vi "UHR-Fleezers Control (host) - 12.1_Jonathan.vi"() -> ()   [LabVIEW 2012] (continued)
      tunnel: w1563 -> [w3002]
      tunnel: w1512 -> [w3001]
      tunnel: w1511 -> [w3000]
      tunnel: w1510 -> [w2999]
      tunnel: w1433 -> [w2998]
      frame #0 {
        n1592 = Or(x="Save N Sets", y="Start Saving") -> (x .or. y?=w2749:bool)
        n1593 = To Double Precision Float(number=w2765) -> (double precision float=w2759:dbl)
        n1594 = Build Array(w2749, "Save Calibration", w2762, w2754) -> (w2764:bool[])
        n1595 = Compound Arithmetic op=OR("Save Calibration", w2762, w2749, w2754) -> (w2767:bool)
        n1596 = Boolean Array To Number(Boolean array=w2764) -> (number=w2761:u32)
        n1597 = feedback #28(FALSE ("Save APD Data\nwith Trap Data")) -> (w2743:bool)
        n1598 = feedback #29(refnum<k0> refnum) -> (w2770:refnum<file>)
        n1599 = feedback #30(refnum<k0> refnum) -> (w2745:refnum<file>)
        n1600 = feedback #31(FALSE ("Save APD Data\nwith Trap Data")) -> (w2753:bool)
        n1601 = feedback #32(refnum<k0> refnum) -> (w2756:refnum<file>)
        n1602 = feedback #33(0) -> (w2772:i32)
        n1603 = feedback #34() -> (w2760:u32)  [unwired: 1 out]
        n1604 = case shown="True" w2767 {
          tunnel: [w2779 1] -> w2768
          tunnel: w2772 -> [w2781 _]
          tunnel: [w2780 w2812] -> w2769
          tunnel: w2770 -> [w2780 _]
          tunnel: w2766 -> [_ w2830]
          tunnel: w2759 -> [_ w2828]
          tunnel: w2761 -> [_ w2831]
          tunnel: [w2778 w2811] -> w2758
          tunnel: w2760 -> [w2778 _]
          tunnel: [w2777 w2809] -> w2755
          tunnel: w2756 -> [w2777 _]
          tunnel: [w2776 w2808] -> w2752
          tunnel: w2753 -> [w2776 _]
          tunnel: "Start Saving" -> [_ w2806]
          tunnel: w2748 -> [_ w2805]
          tunnel: [w2775 w2797] -> w2741
          tunnel: w2745 -> [w2775 _]
          tunnel: [w2774 w2796] -> w2742
          tunnel: w2743 -> [w2774 _]
          frame False {
            n1605 = Increment(x=w2781) -> (x+1=w2779:i32)
          }
          frame True {
            w2802 = FALSE ("Start Saving")
            w2807 = 9.0  # File Version
            w2814 = FALSE ("prepend array or string size? (T)")
            w2813 = T38."big-endian, network order" ("byte order (0:big-endian, network order)")
            n1606 = local read "BD 1 Frequency 1 (MHz)"() -> (w2827:dbl)
            n1607 = local read "BD 2 Frequency 1 (MHz)"() -> (w2826:dbl)
            n1608 = local read "BD 1 Frequency 2 (MHz)"() -> (w2825:dbl)
            n1609 = local read "BD 2 Frequency 2 (MHz)"() -> (w2824:dbl)
            n1610 = local read "BD 1 Frequency 3 (MHz)"() -> (w2823:dbl)
            n1611 = local read "BD 2 Frequency 3 (MHz)"() -> (w2822:dbl)
            n1612 = Array Size(array=w2805) -> (size(s)=w2804:i32)
            n1613 = To Double Precision Float(number=w2804) -> (double precision float=w2803:dbl)
            n1614 = local write "Save Calibration"(w2802) -> ()
            n1615 = local write "Start Saving"(w2802) -> ()
            n1616 = Build Array("Save APD Data\nwith Trap Data", "Save Trap Pos. Data") -> (w2799:bool[])
            n1617 = Boolean Array To Number(Boolean array=w2799) -> (number=w2798:u32)
            n1618 = Build Array(w2827, w2826, w2825, w2824, w2823, w2822) -> (w2821:dbl[])
            n1619 = case shown="1, Default" w2831 {
              tunnel: w2830 -> [w2902 w2922 w2938 w2976]
              tunnel: w2803 -> [w2907 w2929 w2958 w2995]
              tunnel: w2828 -> [w2906 w2928 w2957 w2994]
              tunnel: [w2903 w2924 w2949 w2986] -> w2819
              tunnel: [w2894 "Cal sets to save" w2939 w2977] -> w2811
              tunnel: w2821 -> [w2904 w2925 w2951 w2988]
              tunnel: "Save APD Data\nwith Trap Data" -> [w2901 _ w2935 w2974]
              tunnel: [w2901 w2916 w2935 w2974] -> w2808
              tunnel: w2807 -> [w2897 w2917 w2933 w2972]
              tunnel: w2806 -> [w2896 _ _ _]
              tunnel: [w2887 w2916 w2932 w2962] -> w2796
              tunnel: "Save Trap Pos. Data" -> [w2887 _ w2932 w2962]
              tunnel: w2798 -> [w2886 _ w2931 w2961]
              frame 1, Default {
                # "timeseries"
                n1620 = case shown="True" "Profile" {
                  tunnel: [w2910 w2914] -> w2891
                  tunnel: [w2910 w2913] -> w2890
                  tunnel: [w2910 w2912] -> w2889
                  tunnel: [w2910 w2911] -> w2888
                  frame False {
                    w2910 = 0.0 ("f")
                  }
                  frame True {
                    n1621 = local read "Current Position"() -> (w2915:cluster{dbl, dbl, dbl})
                    n1622 = local read "Y change (mm)"() -> (w2911:dbl)
                    n1623 = Unbundle(w2915) -> (w2914:dbl, w2913:dbl, w2912:dbl)
                  }
                }
                n1624 = local read "Save ave N"() -> (w2909:dbl)
                n1625 = Multiply(x=w2909, y=w2902) -> (x*y=w2908:dbl)
                n1626 = To Double Precision Float(number=w2886) -> (double precision float=w2900:dbl)
                n1627 = Build Array(w2897, w2902, w2908, w2907, w2906, 0.0 ("f")) -> (w2905:dbl[])
                n1628 = Build Array(w2900, w2891, w2890, w2889, w2888) -> (w2898:dbl[])
                n1629 = Select(t=u32 4000000000, s=w2896, f="N sets to save") -> (s? t:f=w2894:u32)
                n1630 = Build Array (concatenate)(w2905, w2904, w2898) -> (w2903:dbl[])
              }
              frame 2 {
                w2919 = 0.0 ("f")
                w2916 = FALSE ("Save APD Data\nwith Trap Data")
                # "calibration"
                n1631 = Boolean To (0,1)(Boolean=w2916) -> (0, 1=w2921:i16)
                n1632 = To Double Precision Float(number=w2921) -> (double precision float=w2920:dbl)
                n1633 = Build Array(w2920, w2919, w2919, w2919, w2919) -> (w2918:dbl[])
                n1634 = Build Array(w2917, w2922, w2922, w2929, w2928, 1.0 ("t")) -> (w2926:dbl[])
                n1635 = Build Array (concatenate)(w2926, w2925, w2918) -> (w2924:dbl[])
                "Calibrating Trap..." <- TRUE ("Calibrating...")
              }
              frame 4 {
                w2936 = 0.0 ("f")
                # "scan dir (x/y = 0/1)"
                # "cycles/step"
                # "n scans (f/b)"
                # "steps"
                # "freq. range"
                # "AOD raster scan"
                n1636 = local read "Number of F/B Scans (AOD)"() -> (w2943:u16)
                n1637 = local read "Cycles/step (AOD)"() -> (w2945:u64)
                n1638 = local read "Scan Range (MHz)"() -> (w2948:dbl)
                n1639 = local read "Scan steps (AOD)"() -> (w2947:u64)
                n1640 = local read "Scan BD"() -> (w2955:bool)
                n1641 = local read "Save ave N"() -> (w2960:dbl)
                n1642 = Boolean To (0,1)(Boolean=w2955) -> (0, 1=w2954:i16)
                n1643 = To Double Precision Float(number=w2943) -> (double precision float=w2942:dbl)
                n1644 = To Double Precision Float(number=w2947) -> (double precision float=w2946:dbl)
                n1645 = To Double Precision Float(number=w2945) -> (double precision float=w2944:dbl)
                n1646 = To Double Precision Float(number=w2954) -> (double precision float=w2953:dbl)
                n1647 = Multiply(x=w2960, y=w2938) -> (x*y=w2959:dbl)
                n1648 = To Double Precision Float(number=w2931) -> (double precision float=w2937:dbl)
                n1649 = Build Array(w2937, w2936, w2936, w2936, w2936) -> (w2934:dbl[])
                n1650 = local read "N sets should be saved"() -> (w2940:dbl)
                n1651 = Build Array(w2953, w2948, w2946, w2944, w2942) -> (w2950:dbl[])
                n1652 = Build Array(w2933, w2938, w2959, w2958, w2957, 2.0 ("t")) -> (w2952:dbl[])
                n1653 = Round Toward +Infinity(x=w2940) -> (ceil(x): smallest int >= x=w2941:dbl)
                n1654 = Build Array (concatenate)(w2952, w2951, w2934, w2950) -> (w2949:dbl[])
                n1655 = To Unsigned Long Integer(number=w2941) -> (unsigned 32bit integer=w2939:u32)
              }
              frame 8 {
                w2969 = 0.0 ("f")
                # "MCL raster scan"
                n1656 = local read "Number of scans (MCL)"() -> (w2964:u64)
                n1657 = local read "Scan lines (y)"() -> (w2963:u64)
                n1658 = local read "2D or 1D Scan"() -> (w2966:bool)
                n1659 = local read "Scan Range (V)\n(of steps)"() -> (w2985:dbl)
                n1660 = local read "Fast Scan Dir"() -> (w2992:bool)
                n1661 = local read "Cycles/step (MCL)"() -> (w2982:u64)
                n1662 = local read "Scan steps (MCL)"() -> (w2984:u64)
                n1663 = Select(t=w2963, s=w2966, f=w2964) -> (s? t:f=w2965:u64)
                n1664 = Boolean To (0,1)(Boolean=w2966) -> (0, 1=w2968:i16)
                n1665 = local read "Save ave N"() -> (w2997:dbl)
                n1666 = local read "Initial X"() -> (w2971:dbl)
                n1667 = local read "Initial Y"() -> (w2970:dbl)
                n1668 = To Double Precision Float(number=w2968) -> (double precision float=w2967:dbl)
                n1669 = Boolean To (0,1)(Boolean=w2992) -> (0, 1=w2991:i16)
                n1670 = To Double Precision Float(number=w2965) -> (double precision float=w2980:dbl)
                n1671 = To Double Precision Float(number=w2984) -> (double precision float=w2983:dbl)
                n1672 = To Double Precision Float(number=w2982) -> (double precision float=w2981:dbl)
                n1673 = To Double Precision Float(number=w2991) -> (double precision float=w2990:dbl)
                n1674 = Multiply(x=w2997, y=w2976) -> (x*y=w2996:dbl)
                n1675 = To Double Precision Float(number=w2961) -> (double precision float=w2975:dbl)
                n1676 = local read "N sets should be saved (MCL)"() -> (w2978:dbl)
                n1677 = Build Array(w2975, w2967, w2969, w2969, w2969) -> (w2973:dbl[])
                n1678 = Build Array(w2990, w2985, w2983, w2981, w2980, w2971, w2970) -> (w2987:dbl[])
                n1679 = Build Array(w2972, w2976, w2996, w2995, w2994, 3.0 ("t")) -> (w2989:dbl[])
                n1680 = Round Toward +Infinity(x=w2978) -> (ceil(x): smallest int >= x=w2979:dbl)
                n1681 = Build Array (concatenate)(w2989, w2988, w2973, w2987) -> (w2986:dbl[])
                n1682 = To Unsigned Long Integer(number=w2979) -> (unsigned 32bit integer=w2977:u32)
              }
            }
            n1683 = local read "Index"() -> (w2836:dbl)
            n1684 = call "Create new save file.vi"("Insert"="", "Ext"=".dat", "Index In"=w2836) -> ("Path Out"=w2794:path, "Index Out"=w2810:dbl)
            n1685 = local write "Save file name"(w2794) -> ()
            n1686 = local write "Index"(w2810) -> ()
            n1687 = local read "connection reference"() -> (w2792:T1)
            n1688 = local write "Save index"(w2810) -> ()
            n1689 = Array Size(array=w2819) -> (size(s)=w2820:i32)
            n1690 = Open/Create/Replace File(file path (use dialog)=w2794, operation (0:open)=T37."create", access (0:read/write)=enum16{"read/write", "read-only", "write-only"}."write-only") -> (refnum out=w2833:refnum<file>)  [unwired: 1 in, 4 out]
            n1691 = local write "Saving..."(TRUE ("Saving...")) -> ()
            n1692 = To Double Precision Float(number=w2820) -> (double precision float=w2818:dbl)
            n1693 = String Length(string="Comment (data description)") -> (length=w2817:i32)
            n1694 = To Double Precision Float(number=w2817) -> (double precision float=w2816:dbl)
            n1695 = Deny Access(7:w2833) -> (3:w2832:refnum<file>)  [unwired: 1 in, 2 out]
            n1696 = Build Array (concatenate)(w2818, w2819, w2816) -> (w2793:dbl[])
            n1697 = case "If fluorescence data to be saved" shown="True" w2808 {
              tunnel: w2794 -> [_ w2885]
              tunnel: [refnum<k0> refnum w2865] -> w2809
              frame False {
              }
              frame True {
                w2864 = 0.0
                n1698 = local read "APD Integration Time (s)"() -> (w2870:dbl)
                n1699 = local read "N APD Samp/step"() -> (w2863:dbl)
                n1700 = Path To String(path=w2885) -> (string=w2884:string)
                n1701 = String Length(string=w2884) -> (length=w2883:i32)
                n1702 = Subtract(x=w2883, y=4) -> (x-y=w2881:i32)
                n1703 = String Subset(string=w2884, length (rest)=w2881) -> (substring=w2880:string)  [unwired: 1 out]
                n1704 = Build Array(w2870, w2863, w2864, w2864, w2864, w2864, w2864, w2864) -> (w2867:dbl[])
                n1705 = Concatenate Strings(w2880, "_fl.dat" ("string")) -> (w2878:string)
                n1706 = Array Size(array=w2867) -> (size(s)=w2869:i32)
                n1707 = String To Path(string=w2878) -> (path=w2874:path)
                n1708 = Open/Create/Replace File(file path (use dialog)=w2874, operation (0:open)=T37."create", access (0:read/write)=enum16{"read/write", "read-only", "write-only"}."write-only") -> (refnum out=w2875:refnum<file>)  [unwired: 1 in, 4 out]
                n1709 = Deny Access(7:w2875) -> (3:w2871:refnum<file>)  [unwired: 1 in, 2 out]
                n1710 = To Double Precision Float(number=w2869) -> (double precision float=w2868:dbl)
                n1711 = Build Array (concatenate)(w2868, w2867) -> (w2866:dbl[])
                n1712 = Write to Binary File(file (use dialog)=w2871, data=w2866, 5:FALSE ("prepend array or string size? (T)"), 9:T38."big-endian, network order" ("byte order (0:big-endian, network order)")) -> (refnum out=w2865:refnum<file>)  [unwired: 1 in, 3 out]
              }
            }
            n1713 = case shown="True" w2796 {
              tunnel: w2794 -> [_ w2847]
              tunnel: [refnum<k0> refnum w2846] -> w2797
              frame False {
              }
              frame True {
                w2842 = 0.0 ("element")
                n1714 = Path To String(path=w2847) -> (string=w2861:string)
                n1715 = Build Array(w2842, w2842, w2842, w2842, w2842, w2842, w2842, w2842) -> (w2843:dbl[])
                n1716 = String Length(string=w2861) -> (length=w2860:i32)
                n1717 = Subtract(x=w2860, y=4) -> (x-y=w2858:i32)
                n1718 = Array Size(array=w2843) -> (size(s)=w2845:i32)
                n1719 = String Subset(string=w2861, length (rest)=w2858) -> (substring=w2857:string)  [unwired: 1 out]
                n1720 = To Double Precision Float(number=w2845) -> (double precision float=w2844:dbl)
                n1721 = Concatenate Strings(w2857, "_pos.dat" ("string")) -> (w2855:string)
                n1722 = Build Array (concatenate)(w2844, w2843) -> (w2841:dbl[])
                n1723 = String To Path(string=w2855) -> (path=w2851:path)
                n1724 = Open/Create/Replace File(file path (use dialog)=w2851, operation (0:open)=T37."create", access (0:read/write)=enum16{"read/write", "read-only", "write-only"}."write-only") -> (refnum out=w2852:refnum<file>)  [unwired: 1 in, 4 out]
                n1725 = Deny Access(7:w2852) -> (3:w2848:refnum<file>)  [unwired: 1 in, 2 out]
                n1726 = Write to Binary File(file (use dialog)=w2848, data=w2841, 5:FALSE ("prepend array or string size? (T)"), 9:T38."big-endian, network order" ("byte order (0:big-endian, network order)")) -> (refnum out=w2846:refnum<file>)  [unwired: 1 in, 3 out]
              }
            }
            n1727 = Write to Binary File(file (use dialog)=w2832, data=w2793, 5:w2814, 9:w2813) -> (refnum out=w2815:refnum<file>)  [unwired: 1 in, 3 out]
            n1728 = Write to Binary File(file (use dialog)=w2815, data="Comment (data description)", 5:w2814, 9:w2813) -> (refnum out=w2812:refnum<file>)  [unwired: 1 in, 3 out]
            n1729 = Bundle("Comment (data description)"="Comment (data description)", "Channel 1 Buffer"="Channel 1 Buffer", "Channel 2 Buffer"="Channel 2 Buffer", "Channel 3 Buffer"="Channel 3 Buffer", "Title"="Title", "DNA Construct"="DNA Construct", "Bead diameter"="Bead diameter", "Name"="Name") -> (w2782:T47)  [unwired: 1 in]
            n1730 = call "MattFileCreator-v9.vi"("Comments"=w2782, "Input Array"=w2793, "File path"=w2794, "table"="labview", "connection reference"=w2792) -> ("connection reference out"=w2791:T1)  [unwired: 5 in, 1 out]
            n1731 = local write "connection reference"(w2791) -> ()
          }
        }
        n1732 = feedback-in #28(w2742) -> ()
        n1733 = feedback-in #29(w2769) -> ()
        n1734 = feedback-in #30(w2741) -> ()
        n1735 = feedback-in #31(w2752) -> ()
        n1736 = feedback-in #32(w2755) -> ()
        n1737 = feedback-in #33(w2768) -> ()
        n1738 = feedback-in #34(w2758) -> ()
      }
      frame #1 {
        n1739 = local read "Saving..."() -> (w3011:bool)
        n1740 = case shown="True" w3011 {
          tunnel: w3015 -> [_ w3026]
          tunnel: w3014 -> [_ w3040]
          tunnel: w3013 -> [_ w3036]
          tunnel: w3012 -> [_ w3035]
          tunnel: w3010 -> [_ w3034]
          tunnel: w3009 -> [_ w3029]
          tunnel: w3008 -> [_ w3028]
          tunnel: w3007 -> [_ w3027]
          tunnel: w3006 -> [_ w3025]
          tunnel: w3005 -> [_ w3023]
          tunnel: w3004 -> [_ w3022]
          tunnel: w3003 -> [_ w3021]
          tunnel: w3002 -> [_ w3020]
          tunnel: w3001 -> [_ w3019]
          tunnel: w3000 -> [_ w3018]
          tunnel: w2999 -> [_ w3017]
          tunnel: w2998 -> [_ w3016]
          frame False {
          }
          frame True {
            n1741 = Multiply(x=w3026, y=w3025) -> (x*y=→"Time (s)":dbl)
            n1742 = Less Or Equal?(x=w3026, y=w3034) -> (x <= y?=w3038:bool)
            n1743 = Or(x="Stop Saving", y="Abort save 2") -> (x .or. y?=w3030:bool)
            n1744 = Not(x=w3030) -> (.not. x?=w3039:bool)
            n1745 = And(x=w3038, y=w3039) -> (x .and. y?=w3037:bool)
            n1746 = case shown="True" w3037 {
              tunnel: w3040 -> [w3047 w3122]
              tunnel: [0.0 w3125] -> w3033
              tunnel: w3026 -> [_ w3123]
              tunnel: w3034 -> [_ w3124]
              tunnel: w3036 -> [_ w3119]
              tunnel: w3035 -> [_ _]
              tunnel: w3029 -> [w3045 w3112]
              tunnel: w3028 -> [w3044 w3113]
              tunnel: w3027 -> [_ w3111]
              tunnel: w3023 -> [_ w3110]
              tunnel: w3022 -> [_ w3054]
              tunnel: w3021 -> [_ w3103]
              tunnel: w3020 -> [_ w3081]
              tunnel: w3019 -> [w3041 w3063]
              tunnel: w3018 -> [w3042 w3062]
              tunnel: w3017 -> [_ w3059]
              tunnel: w3016 -> [_ w3057]
              frame False {
                w3043 = FALSE
                n1747 = Close File(refnum=w3047) -> ()  [unwired: 1 in, 2 out]
                n1748 = case shown="True" w3044 {
                  tunnel: w3045 -> [_ w3049]
                  frame False {
                  }
                  frame True {
                    n1749 = Close File(refnum=w3049) -> ()  [unwired: 1 in, 2 out]
                  }
                }
                n1750 = case shown="True" w3041 {
                  tunnel: w3042 -> [_ w3048]
                  frame False {
                  }
                  frame True {
                    n1751 = Close File(refnum=w3048) -> ()  [unwired: 1 in, 2 out]
                  }
                }
                n1752 = local write "Raster Scanning..."(w3043) -> ()
                n1753 = local write "Calibrating Trap..."(w3043) -> ()
                n1754 = call <vilib>:"Beep.vi"() -> ()  [unwired: 3 in, 9 out]
                n1755 = local write "Stop Saving"(w3043) -> ()
                "Saving..." <- w3043
              }
              frame True {
                n1756 = local read "Calibrating Trap..."() -> (w3114:bool)
                n1757 = case "Write fl. data" shown="True" w3113 {
                  tunnel: w3112 -> [_ w3148]
                  tunnel: w3111 -> [_ w3147]
                  frame False {
                  }
                  frame True {
                    n1758 = Write to Binary File(file (use dialog)=w3148, data=w3147, 5:FALSE ("prepend array or string size? (T)"), 9:T38."big-endian, network order" ("byte order (0:big-endian, network order)")) -> ()  [unwired: 1 in, 4 out]
                  }
                }
                n1759 = Greater?(x="Save ave N", y=1.0) -> (0:w3117:bool)
                n1760 = Not(x=w3114) -> (.not. x?=w3116:bool)
                n1761 = And(x=w3116, y=w3117) -> (x .and. y?=w3060:bool)
                n1762 = case shown="True" w3060 {
                  tunnel: w3059 -> [w3128 w3139]
                  tunnel: [w3128 w3131] -> w3058
                  tunnel: "Save ave N" -> [_ w3132]
                  frame False {
                  }
                  frame True {
                    w3129 = 2 ("dimension size")
                    n1763 = Array Size(array=w3139) -> (size(s)=w3133:i32)
                    n1764 = Divide(x=w3133, y=w3129) -> (x/y=w3137:dbl)
                    n1765 = Reshape Array(w3139, w3137, w3129) -> (w3138:u64[][])
                    n1766 = Transpose 2D Array(2D array=w3138) -> (transposed array=w3136:u64[][])
                    n1767 = for {
                      tunnel: w3136 -> [w3141] mode=indexing
                      tunnel: [w3140] -> w3130 mode=indexing
                      tunnel: w3132 -> [w3142]
                      workers-P: _ -> [_]
                      n1768 = call "downsample 1D array - U64.vi"("Ave N"=w3142, "Array In"=w3141) -> ("Array Out"=w3140:u64[])  [unwired: 1 in]
                    }
                    n1769 = Transpose 2D Array(2D array=w3130) -> (transposed array=w3135:u64[][])
                    n1770 = Divide(x=w3133, y=w3132) -> (x/y=w3134:dbl)
                    n1771 = Reshape Array(w3135, w3134) -> (w3131:u64[])
                  }
                }
                n1772 = case shown="True" w3060 {
                  tunnel: w3119 -> [w3151 w3163]
                  tunnel: [w3151 w3155] -> w3115
                  tunnel: "Save ave N" -> [_ w3156]
                  tunnel: w3110 -> [_ w3154]
                  frame False {
                  }
                  frame True {
                    n1773 = Array Size(array=w3163) -> (size(s)=w3157:i32)
                    n1774 = Array Size(array=w3154) -> (size(s)=w3153:i32)
                    n1775 = Divide(x=w3157, y=w3153) -> (x/y=w3161:dbl)
                    n1776 = Reshape Array(w3163, w3161, w3153) -> (w3162:i16[][])
                    n1777 = Transpose 2D Array(2D array=w3162) -> (transposed array=w3160:i16[][])
                    n1778 = for {
                      tunnel: w3160 -> [w3166] mode=indexing
                      tunnel: [w3165] -> w3152 mode=indexing
                      tunnel: w3156 -> [w3164]
                      workers-P: _ -> [_]
                      n1779 = call "downsample 1D array - I16.vi"("Ave N"=w3164, "Array In"=w3166) -> ("Array Out"=w3165:i16[])  [unwired: 1 out]
                    }
                    n1780 = Transpose 2D Array(2D array=w3152) -> (transposed array=w3159:i16[][])
                    n1781 = Divide(x=w3157, y=w3156) -> (x/y=w3158:dbl)
                    n1782 = Reshape Array(w3159, w3158) -> (w3155:i16[])
                  }
                }
                n1783 = Index Array(array=w3081, index=1) -> (element=w3084:waveform(dbl))
                n1784 = Index Array(array=w3081, index=0) -> (element=w3086:waveform(dbl))
                n1785 = Unbundle By Name(w3084) -> ("Y"=w3088:dbl[])
                n1786 = Unbundle By Name(w3086) -> ("Y"=w3096:dbl[])
                n1787 = case "Write trap pos. data" shown="True" w3063 {
                  tunnel: w3062 -> [_ w3144]
                  tunnel: w3058 -> [_ w3143]
                  frame False {
                  }
                  frame True {
                    n1788 = Write to Binary File(file (use dialog)=w3144, data=w3143, 5:FALSE ("prepend array or string size? (T)"), 9:T38."big-endian, network order" ("byte order (0:big-endian, network order)")) -> ()  [unwired: 1 in, 4 out]
                  }
                }
                n1789 = Write to Binary File(file (use dialog)=w3122, data=w3115, 5:FALSE ("prepend array or string size? (T)"), 9:T38."big-endian, network order" ("byte order (0:big-endian, network order)")) -> ()  [unwired: 1 in, 4 out]
                n1790 = feedback #35(w3088) -> (w3090:dbl[])
                n1791 = Build Array (concatenate)(w3090, w3088) -> (w3089:dbl[])
                n1792 = Select(t=w3088, s=w3054, f=w3089) -> (s? t:f=w3074:dbl[])
                n1793 = feedback-in #35(w3074) -> ()
                n1794 = feedback #36(w3096) -> (w3109:dbl[])
                n1795 = Build Array (concatenate)(w3109, w3096) -> (w3108:dbl[])
                n1796 = Select(t=w3096, s=w3054, f=w3108) -> (s? t:f=w3083:dbl[])
                n1797 = feedback-in #36(w3083) -> ()
                n1798 = Divide(x=w3123, y=w3124) -> (x/y=w3126:dbl)
                n1799 = Multiply(x=w3126, y=100.0) -> (x*y=w3125:dbl)
                n1800 = Build Array(w3083, w3074) -> (→"Saved APD":dbl[][])
                n1801 = Array Size(array=w3083) -> (size(s)=w3101:i32)
                n1802 = Unbundle By Name(w3103) -> ("Y"=w3107:dbl[])
                n1803 = Subtract(x=w3101, y="N pts to average") -> (x-y=w3077:i32)
                n1804 = Multiply(x="N pts to average", y=u16 2) -> (x*y=w3078:u16)
                n1805 = Subtract(x=w3101, y=w3078) -> (x-y=w3076:i32)
                n1806 = feedback #37(w3107) -> (w3106:dbl[])
                n1807 = Build Array (concatenate)(w3106, w3107) -> (w3105:dbl[])
                n1808 = Select(t=w3107, s=w3054, f=w3105) -> (s? t:f=w3104:dbl[])
                "Trap Delta Graph" <- w3104
                n1809 = feedback-in #37(w3104) -> ()
                n1810 = Array Subset(array=w3083, index=w3077, length="N pts to average") -> (w3100:dbl[])
                n1811 = Array Subset(array=w3083, index=w3076, length="N pts to average") -> (w3099:dbl[])
                n1812 = Array Subset(array=w3074, index=w3077, length="N pts to average") -> (w3080:dbl[])
                n1813 = Array Subset(array=w3074, index=w3076, length="N pts to average") -> (w3079:dbl[])
                n1814 = Index Array(array=w3057, index=0) -> (element=w3055:waveform(dbl))
                n1815 = call-poly <vilib>:"Mean.vi"("X"=w3100) -> ("mean"=w3098:dbl)  [unwired: 1 out]
                n1816 = call-poly <vilib>:"Mean.vi"("X"=w3080) -> ("mean"=w3073:dbl)  [unwired: 1 out]
                n1817 = call-poly <vilib>:"Mean.vi"("X"=w3099) -> ("mean"=w3097:dbl)  [unwired: 1 out]
                n1818 = call-poly <vilib>:"Mean.vi"("X"=w3079) -> ("mean"=w3072:dbl)  [unwired: 1 out]
                n1819 = Unbundle By Name(w3055) -> ("Y"=w3052:dbl[])
                n1820 = Subtract(x=w3073, y=w3072) -> (x-y=w3064:dbl)
                "Delta Fl. 2" <- w3064
                n1821 = Subtract(x=w3098, y=w3097) -> (x-y=w3095:dbl)
                "Delta Fl. 1" <- w3095
                n1822 = Initialize Array(w3095, 1 ("dimension size")) -> (w3092:dbl[])
                n1823 = Initialize Array(w3064, 1 ("dimension size")) -> (w3069:dbl[])
                n1824 = feedback #38(w3092) -> (w3093:dbl[])
                n1825 = Build Array (concatenate)(w3093, w3092) -> (w3091:dbl[])
                n1826 = feedback #39(w3069) -> (w3070:dbl[])
                n1827 = Build Array (concatenate)(w3070, w3069) -> (w3068:dbl[])
                n1828 = feedback #40(w3052) -> (w3051:dbl[])
                n1829 = Build Array (concatenate)(w3051, w3052) -> (w3053:dbl[])
                n1830 = Select(t=w3052, s=w3054, f=w3053) -> (s? t:f=w3050:dbl[])
                "Saved trap pos" <- w3050
                n1831 = feedback-in #40(w3050) -> ()
                n1832 = Select(t=w3092, s=w3054, f=w3091) -> (s? t:f=w3067:dbl[])
                n1833 = feedback-in #38(w3067) -> ()
                n1834 = Select(t=w3069, s=w3054, f=w3068) -> (s? t:f=w3066:dbl[])
                n1835 = feedback-in #39(w3066) -> ()
                n1836 = Build Array(w3067, w3066) -> (→"Save APD Deriv":dbl[][])
              }
            }
            "Progress" <- w3033
            "Progress 2" <- w3033
          }
        }
      }
    }
    n1837 = Bundle By Name(cluster=w1683, "Green FB Ch 0"=w1682, "Green FB Ch 1"=w1681) -> (w1661:T46)
    "Green FB Signals (V)" <- w1661
    n1838 = Unbundle By Name(w1661) -> ("Green FB Ch 2"=→"Green FB Plot":dbl)
    n1839 = local read "wait to reset values"() -> (w1752:bool)
    n1840 = Not(x=w1750) -> (.not. x?=w1753:bool)
    n1841 = And(x=w1753, y=w1752) -> (x .and. y?=w1754:bool)
    n1842 = case "Part of MCL raster scanning: returns to initial positions after scan done" shown="True" w1754 {
      tunnel: w1467 -> [w2562 w2569]
      tunnel: [w2562 w2568] -> w1756
      tunnel: w1466 -> [w2561 w2567]
      tunnel: [w2561 w2566] -> w1751
      frame False {
      }
      frame True {
        w2577 = 10.0 ("y")
        w2576 = 32767.0 ("y")
        # "to return scan values\nafter a synchronous \nAOM scan"
        n1843 = local read "AO2"() -> (w2570:dbl)
        n1844 = local read "AO1"() -> (w2571:dbl)
        n1845 = local write "wait to reset values"(FALSE ("wait to reset values")) -> ()
        n1846 = Multiply(x=w2571, y=w2576) -> (x*y=w2573:dbl)
        n1847 = Multiply(x=w2570, y=w2576) -> (x*y=w2575:dbl)
        n1848 = Divide(x=w2573, y=w2577) -> (x/y=w2572:dbl)
        n1849 = Divide(x=w2575, y=w2577) -> (x/y=w2574:dbl)
        n1850 = To Word Integer(number=w2572) -> (16bit integer=w2578:i16)
        n1851 = To Word Integer(number=w2574) -> (16bit integer=w2579:i16)
        n1852 = local read "Total Counts (ticks)"() -> (w2563:u32)
        n1853 = xnode "Read/Write Control"("FPGA VI Reference In"=w2569, "error in"=w2567, "AO1"=w2578, "AO2"=w2579, "MCL count"=w2563) -> ("FPGA VI Reference Out"=w2568:T20, "error out"=w2566:errorcluster)
        n1854 = local read "Scan Range (V)\n(of steps)"() -> (w2564:dbl)
        n1855 = property on="Scan Range (V)\n(of steps)" class="DigNum (strict)"("Val(Sgnl)"=w2564) -> ()  [unwired: 2 in, 2 out]
      }
    }
    n1856 = node-c288() -> ()  [unwired: 2 out]
  }
  n1857 = timed-loop "Control parameters (event loop)" {
    tunnel: w8 -> [w3175]
    shift-right: [w3174] -> _
    shift-left: errorcluster {"status"=FALSE, "code"=0, "source"=""} ("error out") -> [w3173]
    tunnel: [w3172] -> _
    timing: w99 -> [_]
    timing-out: [_] -> w98
    tunnel: w71 -> [w3171]
    tunnel: w12 -> [w3170]
    tunnel: w11 -> [w3169]
    tunnel: w10 -> [w3168]
    tunnel: w9 -> [w3167]
    stop <- w3172 stop-if-true
    n1858 = node-c288() -> ()  [unwired: 2 out]
    n1859 = event shown="[40] \"Index\": Value Change" {
      selector: _ -> [_ _ _ _ _ _ _ _ _ _ _ _ _ _ _ _ _ _ _ _ _ _ _ _ _ _ _ _ _ _ _ _ _ _ _ _ _ _ _ _ _ _ _ _ _ _ _ _ _ _ _ _ _ _ _ _ _ _ _ _ _ _ _ _ _ _ _ _ _ _ _ _ _ _ _ _]
      dyn-events: _ -> [_ _ _ _ _ _ _ _ _ _ _ _ _ _ _ _ _ _ _ _ _ _ _ _ _ _ _ _ _ _ _ _ _ _ _ _ _ _ _ _ _ _ _ _ _ _ _ _ _ _ _ _ _ _ _ _ _ _ _ _ _ _ _ _ _ _ _ _ _ _ _ _ _ _ _ _]
      timeout: _ -> [_ _ _ _ _ _ _ _ _ _ _ _ _ _ _ _ _ _ _ _ _ _ _ _ _ _ _ _ _ _ _ _ _ _ _ _ _ _ _ _ _ _ _ _ _ _ _ _ _ _ _ _ _ _ _ _ _ _ _ _ _ _ _ _ _ _ _ _ _ _ _ _ _ _ _ _]
      tunnel: w3175 -> [w3213 _ _ _ w3251 _ w3273 _ _ _ _ w3339 _ _ w3382 w3388 w3393 w3399 w3435 w3453 w3460 _ w3472 w3476 w3487 w3498 w3509 w3520 w3531 w3542 w3569 w3663 w3670 w3708 _ w3743 w3747 w3758 w3762 w3766 _ w3774 _ _ _ _ _ _ _ _ _ _ _ _ _ _ _ _ _ w4152 _ w4169 _ w4176 w4194 _ w4201 w4209 w4224 w4235 w4241 _ w4250 _ w4269 _]
      tunnel: [w3212 _ _ _ w3241 _ w3272 _ _ w3304 _ w3318 _ _ w3381 w3384 w3390 w3396 w3434 w3451 w3459 _ w3470 _ w3481 w3492 w3503 w3514 w3525 w3536 w3567 w3661 w3668 w3706 _ w3741 w3745 w3748 w3760 w3764 _ w3772 _ _ _ _ _ _ _ _ _ _ _ _ _ _ _ _ _ w4150 _ _ _ _ w4191 _ _ _ _ _ _ _ _ _ _ _] -> w3174
      tunnel: w3173 -> [w3211 _ _ _ w3250 _ w3271 _ _ w3304 _ w3338 _ _ w3380 w3383 w3389 w3395 w3433 w3452 w3458 _ w3471 w3475 w3486 w3497 w3508 w3519 w3530 w3541 w3568 w3662 w3669 w3707 _ w3742 w3746 w3757 w3761 w3765 _ w3773 _ _ _ _ _ _ _ _ _ _ _ _ _ _ _ _ _ w4151 _ w4168 _ w4175 w4193 _ w4200 w4208 w4223 w4234 w4240 _ w4249 _ w4268 _]
      tunnel: [_ _ _ _ _ _ _ _ _ w3303 _ _ _ _ _ _ _ _ _ _ _ _ _ _ _ _ _ _ _ _ _ _ _ _ _ _ _ _ _ _ _ _ _ _ _ _ _ _ _ _ _ _ _ _ _ _ _ _ _ _ _ _ _ _ _ _ _ _ _ _ _ _ _ _ _ _] -> w3172
      tunnel: [_ _ _ _ _ _ _ "Round T1 X" _ _ _ _ _ _ _ _ _ _ _ _ _ _ _ _ _ _ _ _ _ _ _ _ _ _ _ _ _ _ _ _ _ _ _ _ _ _ _ _ _ _ _ _ _ _ _ _ _ _ _ _ _ _ _ _ _ _ _ _ _ _ _ _ _ _ _ _] -> _
      tunnel: [_ _ _ "Adjust Scale\nto Mean" _ _ _ _ _ _ _ _ _ _ _ _ _ _ _ _ _ _ "Test ttrig" _ _ _ _ _ _ _ _ _ _ _ _ _ _ _ _ _ _ _ _ _ _ _ _ _ _ "Flush Sample" "Flush Pump 3" "Flush Pump 1" "Clear Volume" _ _ _ _ _ _ _ _ _ _ _ _ _ _ _ _ _ _ _ _ _ _ _] -> _
      tunnel: [_ _ _ _ _ _ _ _ "Round T2 X" _ "Delayed Interlace Start" _ _ _ _ _ _ _ _ _ _ _ _ _ _ _ _ _ _ _ _ _ _ _ _ _ _ _ _ _ _ _ _ _ _ _ _ _ _ _ _ _ _ _ _ _ _ _ _ _ _ _ _ _ _ _ _ _ _ _ _ _ _ _ _ _] -> _
      tunnel: w3171 -> [_ _ _ _ _ _ _ _ _ _ _ _ _ _ _ _ _ _ _ _ _ _ _ _ _ _ _ _ _ _ _ _ _ _ _ _ _ _ _ _ _ _ _ _ _ w3931 w3938 w3945 w3950 w3959 _ _ w4065 _ _ _ _ _ _ _ _ _ _ _ _ _ _ _ _ _ _ _ _ _ _ _]
      tunnel: w3170 -> [_ _ _ _ _ _ _ _ _ _ _ _ _ _ _ _ _ _ _ _ _ _ _ _ _ _ _ _ _ _ _ _ _ _ _ _ _ _ _ _ _ _ _ w3848 _ _ _ _ _ _ w4003 _ _ w4071 _ w4080 _ w4094 _ _ _ _ _ _ _ _ _ _ _ _ _ _ _ _ _ _]
      tunnel: w3169 -> [_ _ _ _ _ _ _ _ _ _ _ _ _ _ _ _ _ _ _ _ _ _ _ _ _ _ _ _ _ _ _ _ _ _ _ _ _ _ _ _ _ _ _ _ _ _ _ _ _ _ _ _ _ _ _ _ _ _ _ _ _ _ _ _ _ _ _ _ _ _ _ _ _ _ _ _]
      tunnel: w3168 -> [_ _ _ _ _ _ _ _ _ _ _ _ _ _ _ _ _ _ _ _ _ _ _ _ _ _ _ _ _ _ _ _ _ _ _ _ _ _ _ _ _ _ w3785 _ _ _ _ _ _ _ _ w4033 _ _ w4076 _ w4087 _ w4119 _ _ _ _ _ _ _ _ _ _ _ _ _ _ _ _ _]
      tunnel: w3167 -> [_ _ _ _ _ _ _ _ _ _ _ _ _ _ _ _ _ _ _ _ _ _ _ _ _ _ _ _ _ _ _ _ _ _ _ _ _ _ _ _ _ _ _ _ _ _ _ _ _ _ _ _ _ _ _ _ _ _ _ _ _ _ _ _ _ _ _ _ _ _ _ _ _ _ _ _]
      event "AI Count (ticks)", "Sets to FIFO (Traps)", "Save ave N", "FPGA Ave.", "# Samples/channel", "N sets to save": Value Change {
        # "So that if 'Save ave N' is updated, the AOD scanning code updates too."
        n1860 = event-data() -> ()  [unwired: 6 out]
        n1861 = local read "AI Count (ticks)"() -> (w3193:u32)
        n1862 = Boolean To (0,1)(Boolean="Sets to FIFO (Traps)") -> (0, 1=w3203:cluster{"Set 1":i16, "Set 2":i16, "Set 3":i16})
        n1863 = xnode "Read/Write Control"("FPGA VI Reference In"=w3213, "error in"=w3211, "ai count"=w3193, "AI1 Sets to FIFO"="Sets to FIFO (Traps)", "N of AI1 Int Acq Sets"="N Acq Sets (Traps + Fl.)") -> ("error out"=w3212:errorcluster)  [unwired: 1 out]
        n1864 = Cluster To Array(cluster=w3203) -> (array=w3202:i16[])
        n1865 = To Unsigned Long Integer(number=w3202) -> (unsigned 32bit integer=w3182:u32[])
        n1866 = local read "Scan steps (AOD)"() -> (w3204:u64)
        n1867 = Multiply(x=w3193, y="N Acq Sets (Traps + Fl.)") -> (x*y=w3191:u32)
        n1868 = Divide(x=40000000.0, y=w3193) -> (x/y=w3185:dbl)
        "AI rate (Hz)" <- w3185
        "Ave. Rate (Hz)" <- w3185
        n1869 = Add Array Elements(numeric array=w3182) -> (sum=w3194:u32)
        "Trap Sets" <- w3194
        n1870 = Reciprocal(x=w3185) -> (1/x=→"Ave. Period (s)":dbl)
        n1871 = property on="Scan steps (AOD)" class="DigNum (strict)"("Val(Sgnl)"=w3204) -> ()  [unwired: 2 in, 2 out]
        n1872 = Divide(x=w3185, y="N Acq Sets (Traps + Fl.)") -> (x/y=w3208:dbl)
        "Data Rate (Hz)" <- w3208
        n1873 = Reciprocal(x=w3208) -> (1/x=→"Data Period (s)":dbl)
        n1874 = local read "Save ave N"() -> (w3207:dbl)
        n1875 = Divide(x=w3208, y=w3207) -> (x/y=w3206:dbl)
        "Save Data Rate (Hz)" <- w3206
        n1876 = Reciprocal(x=w3206) -> (1/x=→"Save Data Period (s)":dbl)
        n1877 = Multiply(x=w3191, y="# Samples/trap") -> (x*y=w3189:u32)
        "Counts/DMA" <- w3189
        n1878 = property on="Trap Disp. Downsample" class="DigNum (strict)"("Maximum"="# Samples/trap") -> ()  [unwired: 2 in, 2 out]
        n1879 = Multiply(x=w3194, y="# Samples/trap") -> (x*y=w3183:u32)
        "# Samples/channel" <- w3183
        n1880 = Multiply(x=w3183, y=u32 8) -> (x*y=→"Trap AI Elements/DMA read":u32)
        n1881 = local read "APD Int. Count"() -> (w3190:u32)
        n1882 = Multiply(x=w3183, y=u32 3) -> (x*y=→"Trap Pos Elements/DMA read":u32)
        n1883 = Divide(x=w3189, y=w3190) -> (x/y=w3180:dbl)
        "APD Samples/FIFO Acq." <- w3180
        n1884 = Divide(x=w3189, y=40000000.0) -> (x/y=w3187:dbl)
        "DMA Update Period (s)" <- w3187
        n1885 = Multiply(x=2.0, y=w3180) -> (x*y=→"APD Elements/DMA read":dbl)
        n1886 = property on="APD Disp. Downsample" class="DigNum (strict)"("Maximum"=w3180) -> ()  [unwired: 2 in, 2 out]
        n1887 = local read "N sets to save"() -> (w3200:u32)
        n1888 = Multiply(x=w3187, y=w3200) -> (x*y=→"Total Time (s) 2":dbl)
        "FPGA Averaging" <- FALSE ("FPGA Averaging")
      }
      event "Remove Offset": Value Change {
        n1889 = event-data() -> ()  [unwired: 7 out]
        n1890 = local write "Remove Offset"(FALSE ("Remove Offset")) -> ()
        n1891 = local read "Bead Mean (nm)"() -> (w3215:dbl)
        n1892 = local read "Offset (nm)"() -> (w3216:dbl)
        n1893 = Add(x=w3215, y=w3216) -> (x+y=w3214:dbl)
        n1894 = local write "Offset (nm)"(w3214) -> ()
        n1895 = disable-structure shown="Disabled" {
          frame Disabled {
            n1896 = local read "Bead Mean (nm)"() -> (w3221:dbl)
            n1897 = Add(y=w3221) -> (x=w3220:dbl, x+y=w3219:dbl)
            n1898 = Subtract(x=w3221, y=w3220) -> (x-y=w3218:dbl)
            n1899 = property on="Bead Separation" class="WFChart (strict)"("YScale.Minimum"=w3218) -> ()  [unwired: 2 in, 2 out]
            n1900 = property on="Bead Separation" class="WFChart (strict)"("YScale.Maximum"=w3219) -> ()  [unwired: 2 in, 2 out]
          }
          frame Enabled {
          }
        }
      }
      event "Detector Type": Value Change {
        n1901 = event-data() -> ()  [unwired: 7 out]
        n1902 = local read "AI labels"() -> (w3222:string[])
        n1903 = property on="High Res. Display" class="Ring (strict)"("Strings []"=w3222) -> ()  [unwired: 2 in, 2 out]
        n1904 = Build Array (concatenate)(w3222, "none") -> (w3223:string[])
        n1905 = property on="FFT 1 Choice 1" class="Ring (strict)"("Strings []"=w3223) -> ()  [unwired: 2 in, 2 out]
        n1906 = property on="FFT 1 Choice 2" class="Ring (strict)"("Strings []"=w3223) -> ()  [unwired: 2 in, 2 out]
        n1907 = property on="FFT 2 Choice 1" class="Ring (strict)"("Strings []"=w3223) -> ()  [unwired: 2 in, 2 out]
        n1908 = property on="FFT 2 Choice 2" class="Ring (strict)"("Strings []"=w3223) -> ()  [unwired: 2 in, 2 out]
        n1909 = Bundle("APD 1", "APD 2") -> (w3226:cluster{string, string})  [unwired: 1 out]
        n1910 = Cluster To Array(cluster=w3226) -> (array=w3224:string[])
        n1911 = Build Array (concatenate)(w3224, w3223) -> (w3228:string[])
        n1912 = Array Size(array=w3228) -> (size(s)=w3229:i32)
        n1913 = property on="Signals to Plot" class="LstBox (strict)"("Item Names"=w3228) -> ()  [unwired: 2 in, 2 out]
        n1914 = property on="Signals to Plot" class="LstBox (strict)"("Number of Rows"=w3229) -> ()  [unwired: 2 in, 2 out]
        n1915 = property on="All Signals" class="WFChart (strict)"("LegNumRows"=w3229) -> ()  [unwired: 2 in, 2 out]
      }
      event "Adjust Scale\nto Mean": Value Change {
        n1916 = event-data() -> ()  [unwired: 7 out]
        n1917 = local read "APD 1 Rate (Hz)"() -> (w3238:dbl)
        n1918 = Multiply(x=1000.0, y="Above (kHz)") -> (x*y=w3236:dbl)
        n1919 = Multiply(x=1000.0, y="Below (kHz)") -> (x*y=w3234:dbl)
        n1920 = Add(x=w3236, y=w3238) -> (x+y=w3231:dbl)
        n1921 = Subtract(x=w3238, y=w3234) -> (x-y=w3232:dbl)
        n1922 = property on="APD Chart" class="WFChart (strict)"("YScale.Minimum"=w3232) -> ()  [unwired: 2 in, 2 out]
        n1923 = property on="APD Chart" class="WFChart (strict)"("YScale.Maximum"=w3231) -> ()  [unwired: 2 in, 2 out]
      }
      event "Phase adj. (AI1)", "+ phase (AI1)", "- phase (AI1)": Value Change {
        n1924 = event-data() -> ()  [unwired: 7 out]
        n1925 = Negate(x="Phase adj. (AI1)") -> (-x=w3248:i16)
        n1926 = Select(t=w3248, s="- phase (AI1)", f="Phase adj. (AI1)") -> (s? t:f=w3247:i16)
        n1927 = xnode "Read/Write Control"("FPGA VI Reference In"=w3251, "error in"=w3250, "Phase count adjustment"=w3247) -> ("FPGA VI Reference Out"=w3246:T20, "error out"=w3245:errorcluster)
        n1928 = Or(x="- phase (AI1)", y="+ phase (AI1)") -> (x .or. y?=w3242:bool)
        n1929 = xnode "Read/Write Control"("FPGA VI Reference In"=w3246, "error in"=w3245, "+ phase"=w3242) -> ("error out"=w3241:errorcluster)  [unwired: 1 out]
      }
      event "Signals to Plot": Double Click {
        w3254 = u32 9868950 ("Color Box")
        n1930 = event-data() -> ("Row"=w3256:i32)  [unwired: 9 out]
        n1931 = property on="All Signals" class="WFChart (strict)"("Active Plot"=w3256) -> (error out=w3267:errorcluster)  [unwired: 2 in, 1 out]
        n1932 = property on="All Signals" class="WFChart (strict)" props=["Plot", "Visible?", "Plot", "Plot Color"](error in=w3267) -> (error out=w3266:errorcluster, "Plot.Visible?"=w3265:bool)  [unwired: 1 in, 2 out]
        n1933 = Select(t=FALSE ("Plot.Visible"), s=w3265, f=TRUE ("Plot.Visible")) -> (s? t:f=w3260:bool)
        n1934 = property on="All Signals" class="WFChart (strict)"(error in=w3266, "Plot.Visible?"=w3260) -> (error out=w3262:errorcluster)  [unwired: 1 in, 1 out]
        n1935 = property on="All Signals" class="WFChart (strict)"(error in=w3262) -> (error out=w3257:errorcluster, "Plot.Plot Color"=w3261:u32)  [unwired: 1 in, 1 out]
        n1936 = property on="Signals to Plot" class="LstBox (strict)"(error in=w3257, "Active Row"=w3256) -> (error out=w3255:errorcluster)  [unwired: 1 in, 1 out]
        n1937 = Select(t=w3261, s=w3260, f=u32 0) -> (s? t:f=w3258:u32)
        n1938 = property on="Signals to Plot" class="LstBox (strict)"(error in=w3255, "CellFontColor"=w3258, "SelColor"=w3254, "CellBG"=w3254, "CellFontSize"=u32 20 ("Active Row:Cell Font:Size"), "CellFontBold"=TRUE ("Active Row:Cell Font:Bold")) -> ()  [unwired: 1 in, 2 out]
      }
      event "BD 1 Frequency 1 (MHz)", "BD 1 Frequency 2 (MHz)", "BD 1 Frequency 3 (MHz)", "BD 2 Frequency 1 (MHz)", "BD 2 Frequency 2 (MHz)", "BD 2 Frequency 3 (MHz)", "Trap Delta (MHz)": Value Change {
        n1939 = event-data() -> ("CtlRef"=w3270:refnum<vi>)  [unwired: 6 out]
        n1940 = control-ref of="Trap Delta (MHz)"() -> (w3269:refnum<vi>)
        n1941 = Equal?(x=w3269, y=w3270) -> (x = y?=w3268:bool)
        n1942 = case shown="False" "Oscillate Set 1" {
          tunnel: w3273 -> [w3293 _]
          tunnel: [w3292 w3296] -> w3272
          tunnel: w3271 -> [w3291 w3296]
          tunnel: w3268 -> [w3276 _]
          frame False {
            n1943 = local read "BD 1 Frequency 2 (MHz)"() -> (w3280:dbl)
            n1944 = local read "BD 1 Frequency 1 (MHz)"() -> (w3278:dbl)
            n1945 = Subtract(x=w3280, y="Trap Delta (MHz)") -> (x-y=w3277:dbl)
            n1946 = Select(t=w3277, s=w3276, f=w3278) -> (s? t:f=w3275:dbl)
            n1947 = local read "Y RF Frequency Limits (MHz)"() -> (w3281:T17)
            n1948 = local read "X RF Frequency Limits (MHz)"() -> (w3282:T17)
            n1949 = local read "BD 1 Frequency 3 (MHz)"() -> (w3294:dbl)
            n1950 = local write "BD 1 Frequency 1 (MHz)"(w3275) -> ()
            n1951 = local read "BD 2 Frequency 1 (MHz)"() -> (w3285:dbl)
            n1952 = local read "BD 2 Frequency 2 (MHz)"() -> (w3284:dbl)
            n1953 = local read "BD 2 Frequency 3 (MHz)"() -> (w3295:dbl)
            n1954 = call "set RF board frequency - interlace.vi"("Board 2 Frequency Limits"=w3281, "Board 1 Frequency Limits"=w3282, "error in"=w3291, "FPGA VI Reference In"=w3293, "Board 2 Frequency 3 (MHz)"=w3295, "Board 1 Frequency 3 (MHz)"=w3294, "Board 2 Frequency 2 (MHz)"=w3284, "Board 2 Frequency 1 (MHz)"=w3285, "Board 1 Frequency 2 (MHz)"=w3280, "Board 1 Frequency 1  (MHz)"=w3275) -> ("error out"=w3292:errorcluster)  [unwired: 1 out]
            n1955 = Subtract(x=w3285, y=w3284) -> (x-y=w3289:dbl)
            n1956 = Subtract(x=w3275, y=w3280) -> (x-y=w3290:dbl)
            n1957 = Square(x=w3289) -> (x^2=w3287:dbl)
            n1958 = Square(x=w3290) -> (x^2=w3288:dbl)
            n1959 = Add(x=w3288, y=w3287) -> (x+y=w3286:dbl)
            n1960 = Square Root(x=w3286) -> (sqrt(x)=w3283:dbl)
            n1961 = local write "Trap Delta (MHz)"(w3283) -> ()
            n1962 = property on="Initial delta (MHz)" class="DigNum (strict)"("Val(Sgnl)"=w3283) -> ()  [unwired: 2 in, 2 out]
          }
          frame True {
          }
        }
      }
      event "Round T1 X": Value Change {
        n1963 = event-data() -> ()  [unwired: 7 out]
        n1964 = local read "BD 1 Frequency 1 (MHz)"() -> (w3299:dbl)
        n1965 = Round To Nearest(number=w3299) -> (nearest integer value=w3298:dbl)
        n1966 = property on="BD 1 Frequency 1 (MHz)" class="DigNum (strict)"("Val(Sgnl)"=w3298) -> ()  [unwired: 2 in, 2 out]
      }
      event "Round T2 X": Value Change {
        n1967 = event-data() -> ()  [unwired: 7 out]
        n1968 = local read "BD 1 Frequency 2 (MHz)"() -> (w3301:dbl)
        n1969 = Round To Nearest(number=w3301) -> (nearest integer value=w3300:dbl)
        n1970 = property on="BD 1 Frequency 2 (MHz)" class="DigNum (strict)"("Val(Sgnl)"=w3300) -> ()  [unwired: 2 in, 2 out]
      }
      event "Stop All": Value Change {
        n1971 = event-data() -> ()  [unwired: 7 out]
        n1972 = local read "Stop All"() -> (w3303:bool)
      }
      event "Delayed Interlace Start": Value Change {
        n1973 = event-data() -> ()  [unwired: 7 out]
        n1974 = flat-sequence {
          frame #0 {
            n1975 = Multiply(x="Delay to Interlace (s)", y=1000.0) -> (x*y=w3306:dbl)
            n1976 = Wait (ms)(milliseconds to wait=w3306) -> ()  [unwired: 1 out]
          }
          frame #1 {
            n1977 = property on="Green laser mode" class="RadioBtnsControl (strict)"("Val(Sgnl)"=enum32{"Laser ON", "Laser OFF", "Interlace"}."Interlace" ("Value (Signaling)")) -> ()  [unwired: 2 in, 2 out]
          }
        }
      }
      event "BD 1 Amplitude 1 (%)", "BD 1 Amplitude 2 (%)", "BD 1 Amplitude 3 (%)", "BD 2 Amplitude 1 (%)", "BD 2 Amplitude 2 (%)", "BD 2 Amplitude 3 (%)", "Trap 1 ON", "Trap 2 ON", "Trap 3 ON", "Feedback On/Off", "All FB On/Off": Value Change {
        w3330 = i16 1 ("f")
        n1978 = event-data() -> ()  [unwired: 7 out]
        n1979 = local write "Trap 1 (ON/OFF)"("Trap 1 ON") -> ()
        n1980 = local write "Trap 2 (ON/OFF)"("Trap 2 ON") -> ()
        n1981 = Boolean To (0,1)(Boolean="Trap 3 ON") -> (0, 1=w3331:i16)
        n1982 = Boolean To (0,1)(Boolean="Trap 1 ON") -> (0, 1=w3332:i16)
        n1983 = Boolean To (0,1)(Boolean="Trap 2 ON") -> (0, 1=w3333:i16)
        n1984 = Select(t=w3333, s="Trap ON/OFF X or Y Amp?", f=w3330) -> (s? t:f=w3328:i16)
        n1985 = Select(t=w3332, s="Trap ON/OFF X or Y Amp?", f=w3330) -> (s? t:f=w3329:i16)
        n1986 = Select(t=w3331, s="Trap ON/OFF X or Y Amp?", f=w3330) -> (s? t:f=w3327:i16)
        n1987 = Select(t=w3330, s="Trap ON/OFF X or Y Amp?", f=w3333) -> (s? t:f=w3325:i16)
        n1988 = Select(t=w3330, s="Trap ON/OFF X or Y Amp?", f=w3332) -> (s? t:f=w3326:i16)
        n1989 = Select(t=w3330, s="Trap ON/OFF X or Y Amp?", f=w3331) -> (s? t:f=w3324:i16)
        n1990 = And(x="All FB On/Off", y="Feedback On/Off") -> (x .and. y?=w3322:cluster{"Set 1":bool, "Set 2":bool})
        n1991 = local read "BD 1 Amplitude 1 (%)"() -> (w3342:dbl)
        n1992 = local read "BD 1 Amplitude 2 (%)"() -> (w3341:dbl)
        n1993 = local read "BD 1 Amplitude 3 (%)"() -> (w3340:dbl)
        n1994 = Unbundle By Name(w3322) -> ("Set 1"=w3317:bool, "Set 2"=w3314:bool)
        n1995 = local read "Y RF Amplitude Limits (%)"() -> (w3310:T17)
        n1996 = local read "X RF Amplitude Limits (%)"() -> (w3311:T17)
        n1997 = local read "BD 2 Amplitude 1 (%)"() -> (w3343:dbl)
        n1998 = local read "BD 2 Amplitude 2 (%)"() -> (w3344:dbl)
        n1999 = local read "BD 2 Amplitude 3 (%)"() -> (w3345:dbl)
        n2000 = And(x="Trap 2 ON", y=w3314) -> (x .and. y?=w3312:bool)
        n2001 = And(x="Trap 1 ON", y=w3317) -> (x .and. y?=w3315:bool)
        n2002 = Multiply(x=w3329, y=w3342) -> (x*y=w3337:dbl)
        n2003 = Multiply(x=w3341, y=w3328) -> (x*y=w3335:dbl)
        n2004 = Multiply(x=w3340, y=w3327) -> (x*y=w3336:dbl)
        n2005 = Multiply(x=w3343, y=w3326) -> (x*y=w3346:dbl)
        n2006 = Multiply(x=w3344, y=w3325) -> (x*y=w3347:dbl)
        n2007 = Multiply(x=w3345, y=w3324) -> (x*y=w3348:dbl)
        n2008 = call "set RF board amplitude - interlace.vi"("Board 2 Amplitude Limits"=w3310, "Board 1 Amplitude Limits"=w3311, "error in"=w3338, "FPGA VI Reference In"=w3339, "Board 2 Amplitude 3 (%)"=w3348, "Board 1 Amplitude 3 (%)"=w3336, "Board 2 Amplitude 2 (%)"=w3347, "Board 2 Amplitude 1 (%)"=w3346, "Board 1 Amplitude 2 (%)"=w3335, "Board 1 Amplitude 1 (%)"=w3337) -> ("error out"=w3319:errorcluster, "FPGA VI Reference Out"=w3320:T20)
        n2009 = xnode "Read/Write Control"("FPGA VI Reference In"=w3320, "error in"=w3319, "FB On/Off Set 1"=w3315, "FB On/Off Set 2"=w3312) -> ("error out"=w3318:errorcluster)  [unwired: 1 out]
      }
      event "Load parameters": Value Change {
        n2010 = event-data() -> ()  [unwired: 7 out]
        n2011 = property on="Saved AOD Raster Scan Parameter Sets" class="Arr (strict)"() -> ("Index Values"=w3359:u32[])  [unwired: 2 in, 2 out]
        n2012 = Index Array(array=w3359, index=0) -> (element=w3356:u32)
        n2013 = local write "Load parameters"(FALSE ("Load parameters")) -> ()
        n2014 = Index Array(array="Saved AOD Raster Scan Parameter Sets", index=w3356) -> (element=w3355:T48)
        n2015 = Unbundle By Name(w3355) -> ("Scan Range AOD (nm) 2"=w3354:dbl, "Step Size AOD (nm) 2"=w3353:dbl, "Scan Speed AOD (nm/s) 2"=w3352:dbl, "Number of scans (AOD) 2"=w3351:u16)
        n2016 = flat-sequence {
          tunnel: w3354 -> [w3362]
          tunnel: w3353 -> [w3361]
          tunnel: w3352 -> [w3360]
          tunnel: w3351 -> [w3363]
          frame #0 {
            n2017 = local write "Scan Speed (nm/s)"(w3360) -> ()
            n2018 = local write "Scan Range (nm)"(w3362) -> ()
            n2019 = local write "Step Size (nm)"(w3361) -> ()
          }
          frame #1 {
            n2020 = property on="Number of F/B Scans (AOD)" class="DigNum (strict)"("Val(Sgnl)"=w3363) -> ()  [unwired: 2 in, 2 out]
          }
        }
      }
      event "Trap 1 (ON/OFF)", "Trap 2 (ON/OFF)": Value Change {
        n2021 = event-data() -> ()  [unwired: 7 out]
        n2022 = property on="Trap 2 ON" class="Bool (strict)"("Val(Sgnl)"="Trap 2 (ON/OFF)") -> ()  [unwired: 2 in, 2 out]
        n2023 = property on="Trap 1 ON" class="Bool (strict)"("Val(Sgnl)"="Trap 1 (ON/OFF)") -> ()  [unwired: 2 in, 2 out]
      }
      event "DIO count 1 (ticks)", "DIO count 2 (ticks)", "DIO count 3 (ticks)", "Interlace", "Number Interlace Sets", "Not-Interlacing Set": Value Change {
        n2024 = event-data() -> ()  [unwired: 7 out]
        n2025 = local read "DIO count 3 (ticks)"() -> (w3376:u32)
        n2026 = local read "DIO count 1 (ticks)"() -> (w3378:u32)
        n2027 = local read "DIO count 2 (ticks)"() -> (w3377:u32)
        n2028 = To Unsigned Byte Integer(number="Not-Interlacing Set") -> (unsigned 8bit integer=w3367:u8)
        n2029 = Add(x=w3367, y=u8 1) -> (x+y=w3371:u8)
        n2030 = xnode "Read/Write Control"("FPGA VI Reference In"=w3382, "error in"=w3380, "DIO count 1 (ticks)"=w3378, "DIO count 2 (ticks)"=w3377, "DIO count 3 (ticks)"=w3376, "Interlace ON/OFF"="Interlace", "Number Interlace Cycles"="Number Interlace Sets", "Interlace Off Parameters"=w3371) -> ("error out"=w3381:errorcluster)  [unwired: 1 out]
        n2031 = Build Array(w3378, w3377, w3376) -> (w3369:u32[])
        n2032 = Split 1D Array(array=w3369, index="Number Interlace Sets") -> (first subarray=w3379:u32[])  [unwired: 1 out]
        n2033 = Index Array(array=w3369, index=w3367) -> (element=w3368:u32)
        n2034 = Add Array Elements(numeric array=w3379) -> (sum=w3373:u32)
        n2035 = Select(t=w3373, s="Interlace", f=w3368) -> (s? t:f=→"Total Counts (ticks)":u32)
      }
      event "Reset Feedback": Value Change {
        n2036 = event-data() -> ()  [unwired: 7 out]
        n2037 = Unbundle By Name("Reset Feedback") -> ("Set 1"=w3386:bool, "Set 2"=w3385:bool)
